vi "voltimetro.vi"() -> ()   [LabVIEW 2012]
uses:
  <vilib>/LabVIEW Interface for Arduino/Type Defs/Analog Pin.ctl
  <vilib>/LabVIEW Interface for Arduino/LabVIEW Interface for Arduino.lvlib
panel:
  out "Voltios":bool
  out "mVoltios":bool
  out "kVoltios":bool
  in  "Ring":u16(ring) caption="Magnitud" items=["mVoltios", "Voltios", "kVoltios"]
  out "Voltímetro kV":dbl(knob) caption="Voltímetro" scale=0.0..0.015
  out "Voltímetro V":dbl(knob) caption="Voltímetro" scale=0.0..10.0
  out "Voltímetro mV":dbl(knob) caption="Voltímetro" scale=0.0..10000.0
  in  "stop":bool
  # "WWW.GEEKYTHEORY.COM"
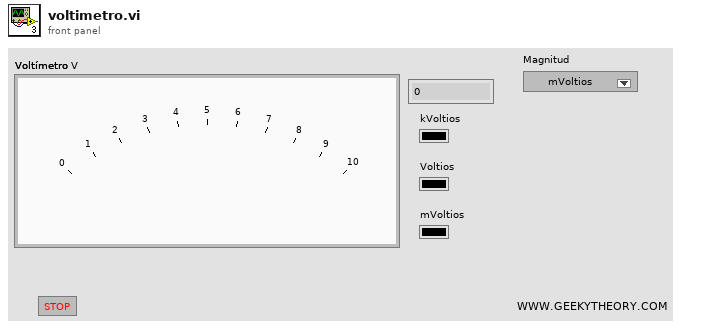
[diagram p1: front panel]
types:
  T1 = typedef "LabVIEW Interface for Arduino.lvlib/Arduino Resource.ctl" = cluster{"VISA resource":refnum<visa-resource-name>, "Board Type":T2, "Connection Type":enum8{"USB / Serial"}, "Bytes Per Packet (15)":u8}
  T2 = typedef "LabVIEW Interface for Arduino.lvlib/Board Type.ctl" = enum16{"Uno", "Dimuelanove w/Atmega 328", "Mega 2560"}
  T3 = typedef "LabVIEW Interface for Arduino.lvlib/Analog Pin.ctl" = enum8{"Anlog In 0", "Anlog In 1", "Anlog In 2", "Anlog In 3", "Anlog In 4", "Anlog In 5"}
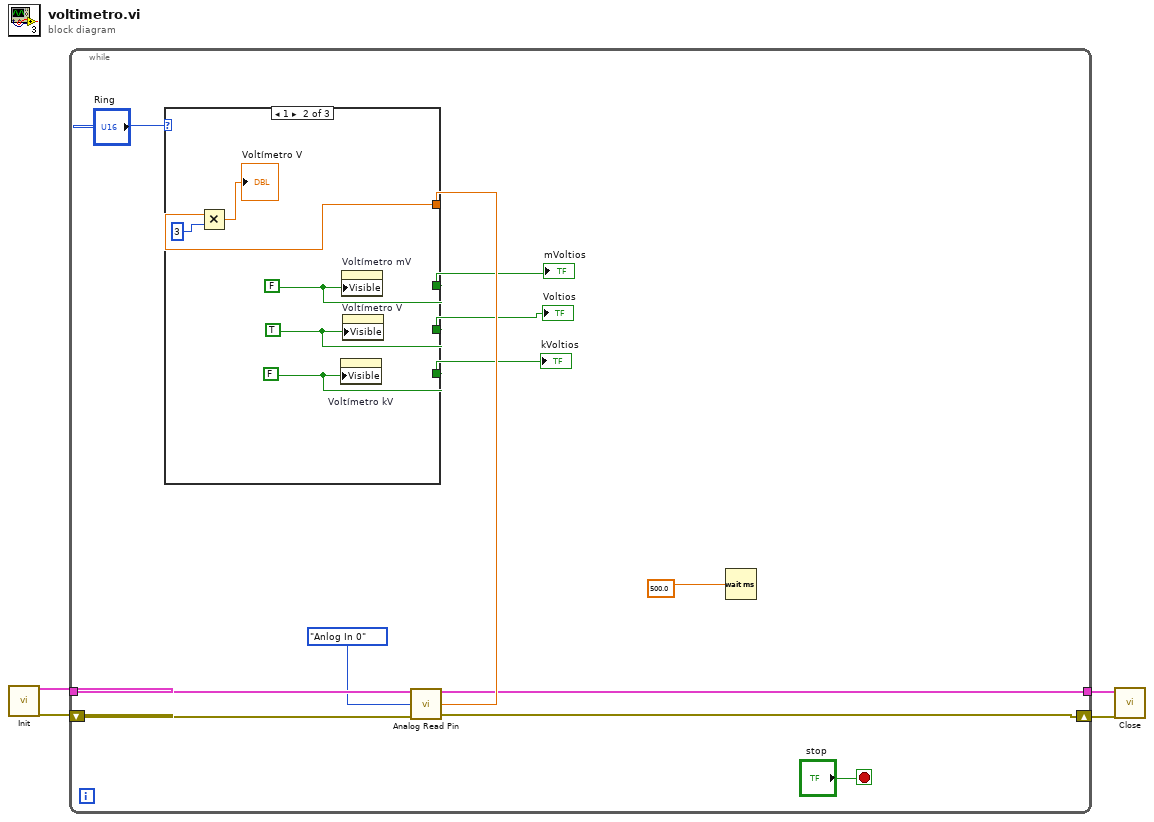
[diagram p0: block diagram]
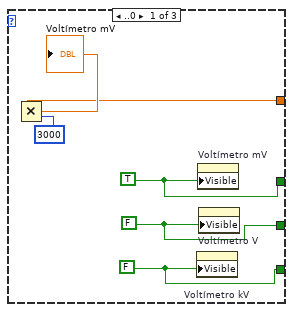
[diagram p2: hidden frame]
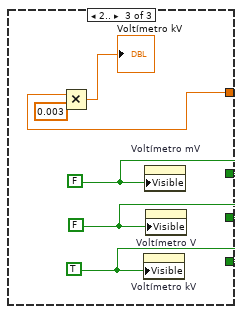
[diagram p3: hidden frame]
diagram:
  n1 = call <vilib>:"Init.vi"() -> ("Arduino Resource"=w4:T1, "error out"=w2:errorcluster)  [unwired: 18 in]
  n2 = while {
    shift-right: [w5] -> w1
    shift-left: w2 -> [w14]
    tunnel: w4 -> [w15]
    tunnel: [w6] -> w3
    stop <- "stop" stop-if-true
    n3 = call <vilib>:"Analog Read Pin.vi"("Arduino Resource"=w15, "Analog Input Pin (0)"=Analog_Pin."Anlog In 0" ("Analog Pin"), "error in"=w14) -> ("Arduino Resource"=w6:T1, "Voltage"=w12:dbl, "error out"=w5:errorcluster)  [unwired: 10 in]
    n4 = case shown="1" "Ring" {
      tunnel: w12 -> [w20 w26 w32]
      tunnel: [w19 w25 w31] -> w10
      tunnel: [w18 w24 w30] -> w9
      tunnel: [w17 w23 w29] -> w8
      frame ..0 {
        w19 = TRUE
        w17 = FALSE
        w18 = FALSE
        n5 = Multiply(x=w20, y=3000) -> (x*y=→"Voltímetro mV":dbl)
        n6 = property on="Voltímetro kV" class="Knob (strict)"("Visible"=w17) -> ()  [unwired: 2 in, 2 out]
        n7 = property on="Voltímetro mV" class="Knob (strict)"("Visible"=w19) -> ()  [unwired: 2 in, 2 out]
        n8 = property on="Voltímetro V" class="Knob (strict)"("Visible"=w18) -> ()  [unwired: 2 in, 2 out]
      }
      frame 1 {
        w25 = FALSE
        w23 = FALSE
        w24 = TRUE
        n9 = Multiply(x=w26, y=3) -> (x*y=→"Voltímetro V":dbl)
        n10 = property on="Voltímetro kV" class="Knob (strict)"("Visible"=w23) -> ()  [unwired: 2 in, 2 out]
        n11 = property on="Voltímetro mV" class="Knob (strict)"("Visible"=w25) -> ()  [unwired: 2 in, 2 out]
        n12 = property on="Voltímetro V" class="Knob (strict)"("Visible"=w24) -> ()  [unwired: 2 in, 2 out]
      }
      frame 2.. {
        w31 = FALSE
        w29 = TRUE
        w30 = FALSE
        n13 = Multiply(x=w32, y=0.003) -> (x*y=→"Voltímetro kV":dbl)
        n14 = property on="Voltímetro kV" class="Knob (strict)"("Visible"=w29) -> ()  [unwired: 2 in, 2 out]
        n15 = property on="Voltímetro mV" class="Knob (strict)"("Visible"=w31) -> ()  [unwired: 2 in, 2 out]
        n16 = property on="Voltímetro V" class="Knob (strict)"("Visible"=w30) -> ()  [unwired: 2 in, 2 out]
      }
    }
    "kVoltios" <- w8
    "mVoltios" <- w10
    "Voltios" <- w9
    n17 = Wait (ms)(milliseconds to wait=500.0) -> ()  [unwired: 1 out]
  }
  n18 = call <vilib>:"Close.vi"("Arduino Resource"=w3, "error in"=w1) -> ()  [unwired: 13 in, 1 out]
